vi "Parse CLI Arguments.vi"(4 "error in":errorcluster, 7 "CLI Data in":T1) -> (0 "error out":errorcluster, 3 "CLI Data out":T1)   [LabVIEW 2025]
doc: "Parse CLI parameters and flags."
uses:
  Type Definitions/CLI Data--cluster.ctl
  <vilib>/Wiresmith Technology/G CLI/CLI Class/CLI.lvclass
  <vilib>/Wiresmith Technology/G CLI/Argument Parser/Option Set Class/Option Set.lvclass
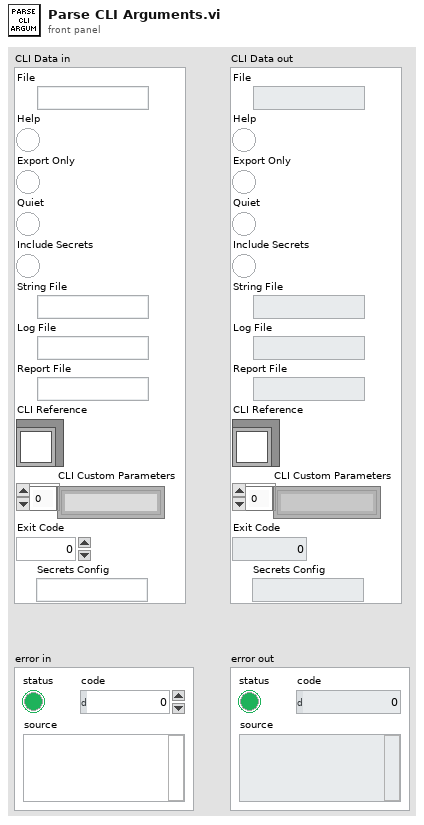
[diagram p1: front panel]
types:
  T1 = typedef "CLI Data--cluster.ctl" = cluster{"File":path, "Help":bool, "Export Only":bool, "Quiet":bool, "Include Secrets":bool, "String File":path, "Log File":path, "Report File":path, "CLI Reference":refnum<class "CLI.lvclass">, "CLI Custom Parameters":string[], "Exit Code":i32, "Secrets Config":path}
  T2 = typedef "Option Parser.lvlib/Option.lvclass/Option Configuration.ctl" = cluster{"Option Type":T3, "Option Labels":string[], "Key":string, "Description":string, "Required":bool, "Default Value":string}
  T3 = typedef "Option Parser.lvlib/Option.lvclass/Argument Type.ctl" = enum16{"flag", "value"}
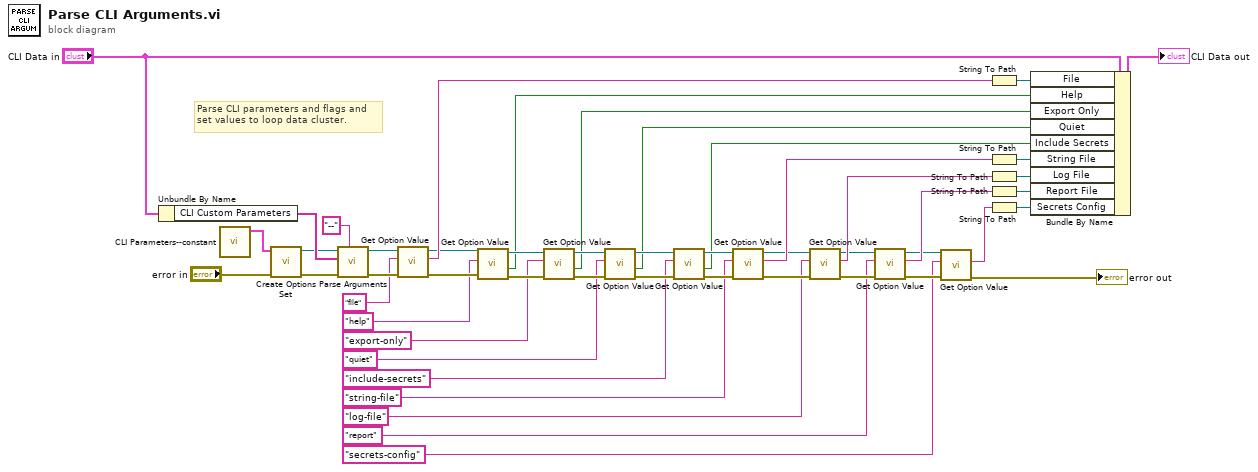
[diagram p0: block diagram]
diagram:
  # "Parse CLI parameters and flags and\nset values to loop data cluster."
  n1 = Unbundle By Name("CLI Data in") -> ("CLI Custom Parameters"=w38:string[])
  n2 = call "CLI Parameters--constant.vi"() -> ("CLI Parameters"=w33:T2[])  [unwired: 7 in]
  n3 = call <vilib>:"Create Options Set.vi"("error in (no error)"="error in", "Options"=w33) -> ("error out"=w49:errorcluster, "Option Set out"=w34:refnum<class "Option Set.lvclass">)  [unwired: 8 in]
  n4 = call <vilib>:"Parse Arguments.vi"("Label Marker (-)"="--", "error in (no error)"=w49, "Arguments"=w38, "Option Set in"=w34) -> ("error out"=w48:errorcluster, "Option Set out"=w18:refnum<class "Option Set.lvclass">)  [unwired: 4 in, 2 out]
  n5 = call <vilib>:"Get Option Value.vi"("error in (no error)"=w48, "Option Key"="file", "Option Set in"=w18) -> ("error out"=w47:errorcluster, "Value"=w31:string, "Option Set out"=w17:refnum<class "Option Set.lvclass">)  [unwired: 5 in, 1 out]
  n6 = call <vilib>:"Get Option Value.vi"("error in (no error)"=w47, "Option Key"="help", "Option Set in"=w17) -> ("error out"=w46:errorcluster, "Set"=w2:bool, "Option Set out"=w16:refnum<class "Option Set.lvclass">)  [unwired: 5 in, 1 out]
  n7 = call <vilib>:"Get Option Value.vi"("error in (no error)"=w46, "Option Key"="export-only", "Option Set in"=w16) -> ("error out"=w45:errorcluster, "Set"=w3:bool, "Option Set out"=w15:refnum<class "Option Set.lvclass">)  [unwired: 5 in, 1 out]
  n8 = call <vilib>:"Get Option Value.vi"("error in (no error)"=w45, "Option Key"="quiet", "Option Set in"=w15) -> ("error out"=w44:errorcluster, "Set"=w4:bool, "Option Set out"=w14:refnum<class "Option Set.lvclass">)  [unwired: 5 in, 1 out]
  n9 = call <vilib>:"Get Option Value.vi"("error in (no error)"=w44, "Option Key"="include-secrets", "Option Set in"=w14) -> ("error out"=w43:errorcluster, "Set"=w5:bool, "Option Set out"=w13:refnum<class "Option Set.lvclass">)  [unwired: 5 in, 1 out]
  n10 = call <vilib>:"Get Option Value.vi"("error in (no error)"=w43, "Option Key"="string-file", "Option Set in"=w13) -> ("error out"=w42:errorcluster, "Value"=w25:string, "Option Set out"=w12:refnum<class "Option Set.lvclass">)  [unwired: 5 in, 1 out]
  n11 = call <vilib>:"Get Option Value.vi"("error in (no error)"=w42, "Option Key"="log-file", "Option Set in"=w12) -> ("error out"=w41:errorcluster, "Value"=w23:string, "Option Set out"=w11:refnum<class "Option Set.lvclass">)  [unwired: 5 in, 1 out]
  n12 = call <vilib>:"Get Option Value.vi"("error in (no error)"=w41, "Option Key"="report", "Option Set in"=w11) -> ("error out"=w40:errorcluster, "Value"=w21:string, "Option Set out"=w10:refnum<class "Option Set.lvclass">)  [unwired: 5 in, 1 out]
  n13 = call <vilib>:"Get Option Value.vi"("error in (no error)"=w40, "Option Key"="secrets-config", "Option Set in"=w10) -> ("error out"=→"error out":errorcluster, "Value"=w19:string)  [unwired: 5 in, 2 out]
  n14 = String To Path(string=w31) -> (path=w1:path)
  n15 = String To Path(string=w25) -> (path=w6:path)
  n16 = String To Path(string=w23) -> (path=w7:path)
  n17 = String To Path(string=w21) -> (path=w8:path)
  n18 = String To Path(string=w19) -> (path=w9:path)
  n19 = Bundle By Name(cluster="CLI Data in", "File"=w1, "Help"=w2, "Export Only"=w3, "Quiet"=w4, "Include Secrets"=w5, "String File"=w6, "Log File"=w7, "Report File"=w8, "Secrets Config"=w9) -> (→"CLI Data out":T1)
